vi "Receiver_Example - 1 Channel_Control.vi"() -> ()   [LabVIEW 2022 SP3]
panel:
  out "Numeric":dbl
  out "Iterations 2":i32
  in  "OFDM - 4QAM/16QAM":bool
  out "Error out 2":errorcluster
  in  "Tab Control 2":enum32{"OFDM - 4QAM", "16QAM"}(tab)
  in  "Tab Control":enum32{"USRP Parameters", "Rx Info", "BER"}(tab)
  in  "USRP ControledParameters":T1={"Active Antenna"="RX2", "Gain (dB)"=10.0, "Carrier Frequency"=2400000000.0, "IQ Rate"=2000000.0, "Active channels"="0"} {"IQ Rate" format="%#_6p"; "Carrier Frequency" format="%#_6p"; "Gain (dB)" format="%#_6f"}
  in  "Device selection":refnum<k15>="RIO0"
  in  "Trigger level":dbl=0.005 format="%f"
  out "?":T2
  out "SIG valid?":bool
  out "Frequency offset":dbl
  out "Coerced Parameters":T3={"IQ Rate"=100000.0, "Carrier  Freq."=100000.0, "Gain"=0.0} {"Gain" format="%#_6f"; "Carrier  Freq." format="%#_6p"; "IQ Rate" format="%#_6p"}
  out "Error out":errorcluster
  in  "Boolean":bool
  in  "Expected message LP":string="Non Critical Data\nNon Critical Data\nNon Critical Data\nNon Critical Data\nNon Critical Data"
  in  "Record BER":bool
  in  "Refresh Button":bool
  out "Inst. BER LP":dbl format="%#_4g"
  out "No. Bits LP":dbl
  out "Acum. Err LP":dbl
  out "Acc. BER LP":dbl format="%#_4g"
  in  "Expected message 2 HP":string="Critical Dataaaaa\nCritical Dataaaaa\nCritical Dataaaaa\nCritical Dataaaaa\nCritical Dataaaaa"
  out "Inst. BER HP":dbl format="%#_4g"
  out "Acum. Err HP":dbl
  out "No. Bits HP":dbl
  out "Acc. BER  HP":dbl format="%#_4g"
  out "Expected message LP Detected":string="Non Critical Data\nNon Critical Data\nNon Critical Data\nNon Critical Data\nNon Critical Data"
  out "Expected message  HP  Detected":string="Critical Dataaaaa\nCritical Dataaaaa\nCritical Dataaaaa\nCritical Dataaaaa\nCritical Dataaaaa"
  in  "Boolean 2":bool
  out "Constellation Map":cdb[](graph)
  out "Low-Power Decoded Message":string
  out "High-Power Decoded Message":string
  out "Low-Power BER Graph":dbl(graph)
  out "High-Power BER Graph":dbl(graph)
  out "Low-Power Instantaneous BER Graph":u8(slide) scale=0.0..100.0
  out "High-Power Instantaneous BER Graph":u8(slide) scale=0.0..100.0
  in  "Low-Power Window Size":dbl=15.0 format="%#_6p"
  in  "High-Power Window Size":dbl=15.0 format="%#_6p"
  out "Reconstructed Image":T4(plugin-control)
  out "Expected message  HP  Detected 2":string="Critical Dataaaaa\nCritical Dataaaaa\nCritical Dataaaaa\nCritical Dataaaaa\nCritical Dataaaaa"
  in  "Boolean 3":bool
  in  "High-Power Window Size 2":dbl=15.0 format="%#_6p"
  out "High-Power Instantaneous BER Graph 2":u8(slide) scale=0.0..100.0
  out "High-Power BER Graph 2":dbl(graph)
  out "No. Bits HP 2":dbl
  out "Acc. BER  HP 2":dbl format="%#_4g"
  out "Acum. Err HP 2":dbl
  out "Inst. BER HP 2":dbl format="%#_4g"
  in  "Expected message 2 HP 2":string="Critical Dataaaaa\nCritical Dataaaaa\nCritical Dataaaaa\nCritical Dataaaaa\nCritical Dataaaaa"
  out "High-Power Decoded Message 2":string
  in  "Record BER 2":bool
  out "Constellation Map 2":cdb[](graph)
  out "Frequency offset 2":dbl
  out "SIG valid? 2":bool
  in  "Refresh Button 2":bool
  out "Reconstructed Image":T4(plugin-control)
  out "Iterations":i32
  in  "error in (no error)":errorcluster
  # "OFDM Superposition Coded Receiver"
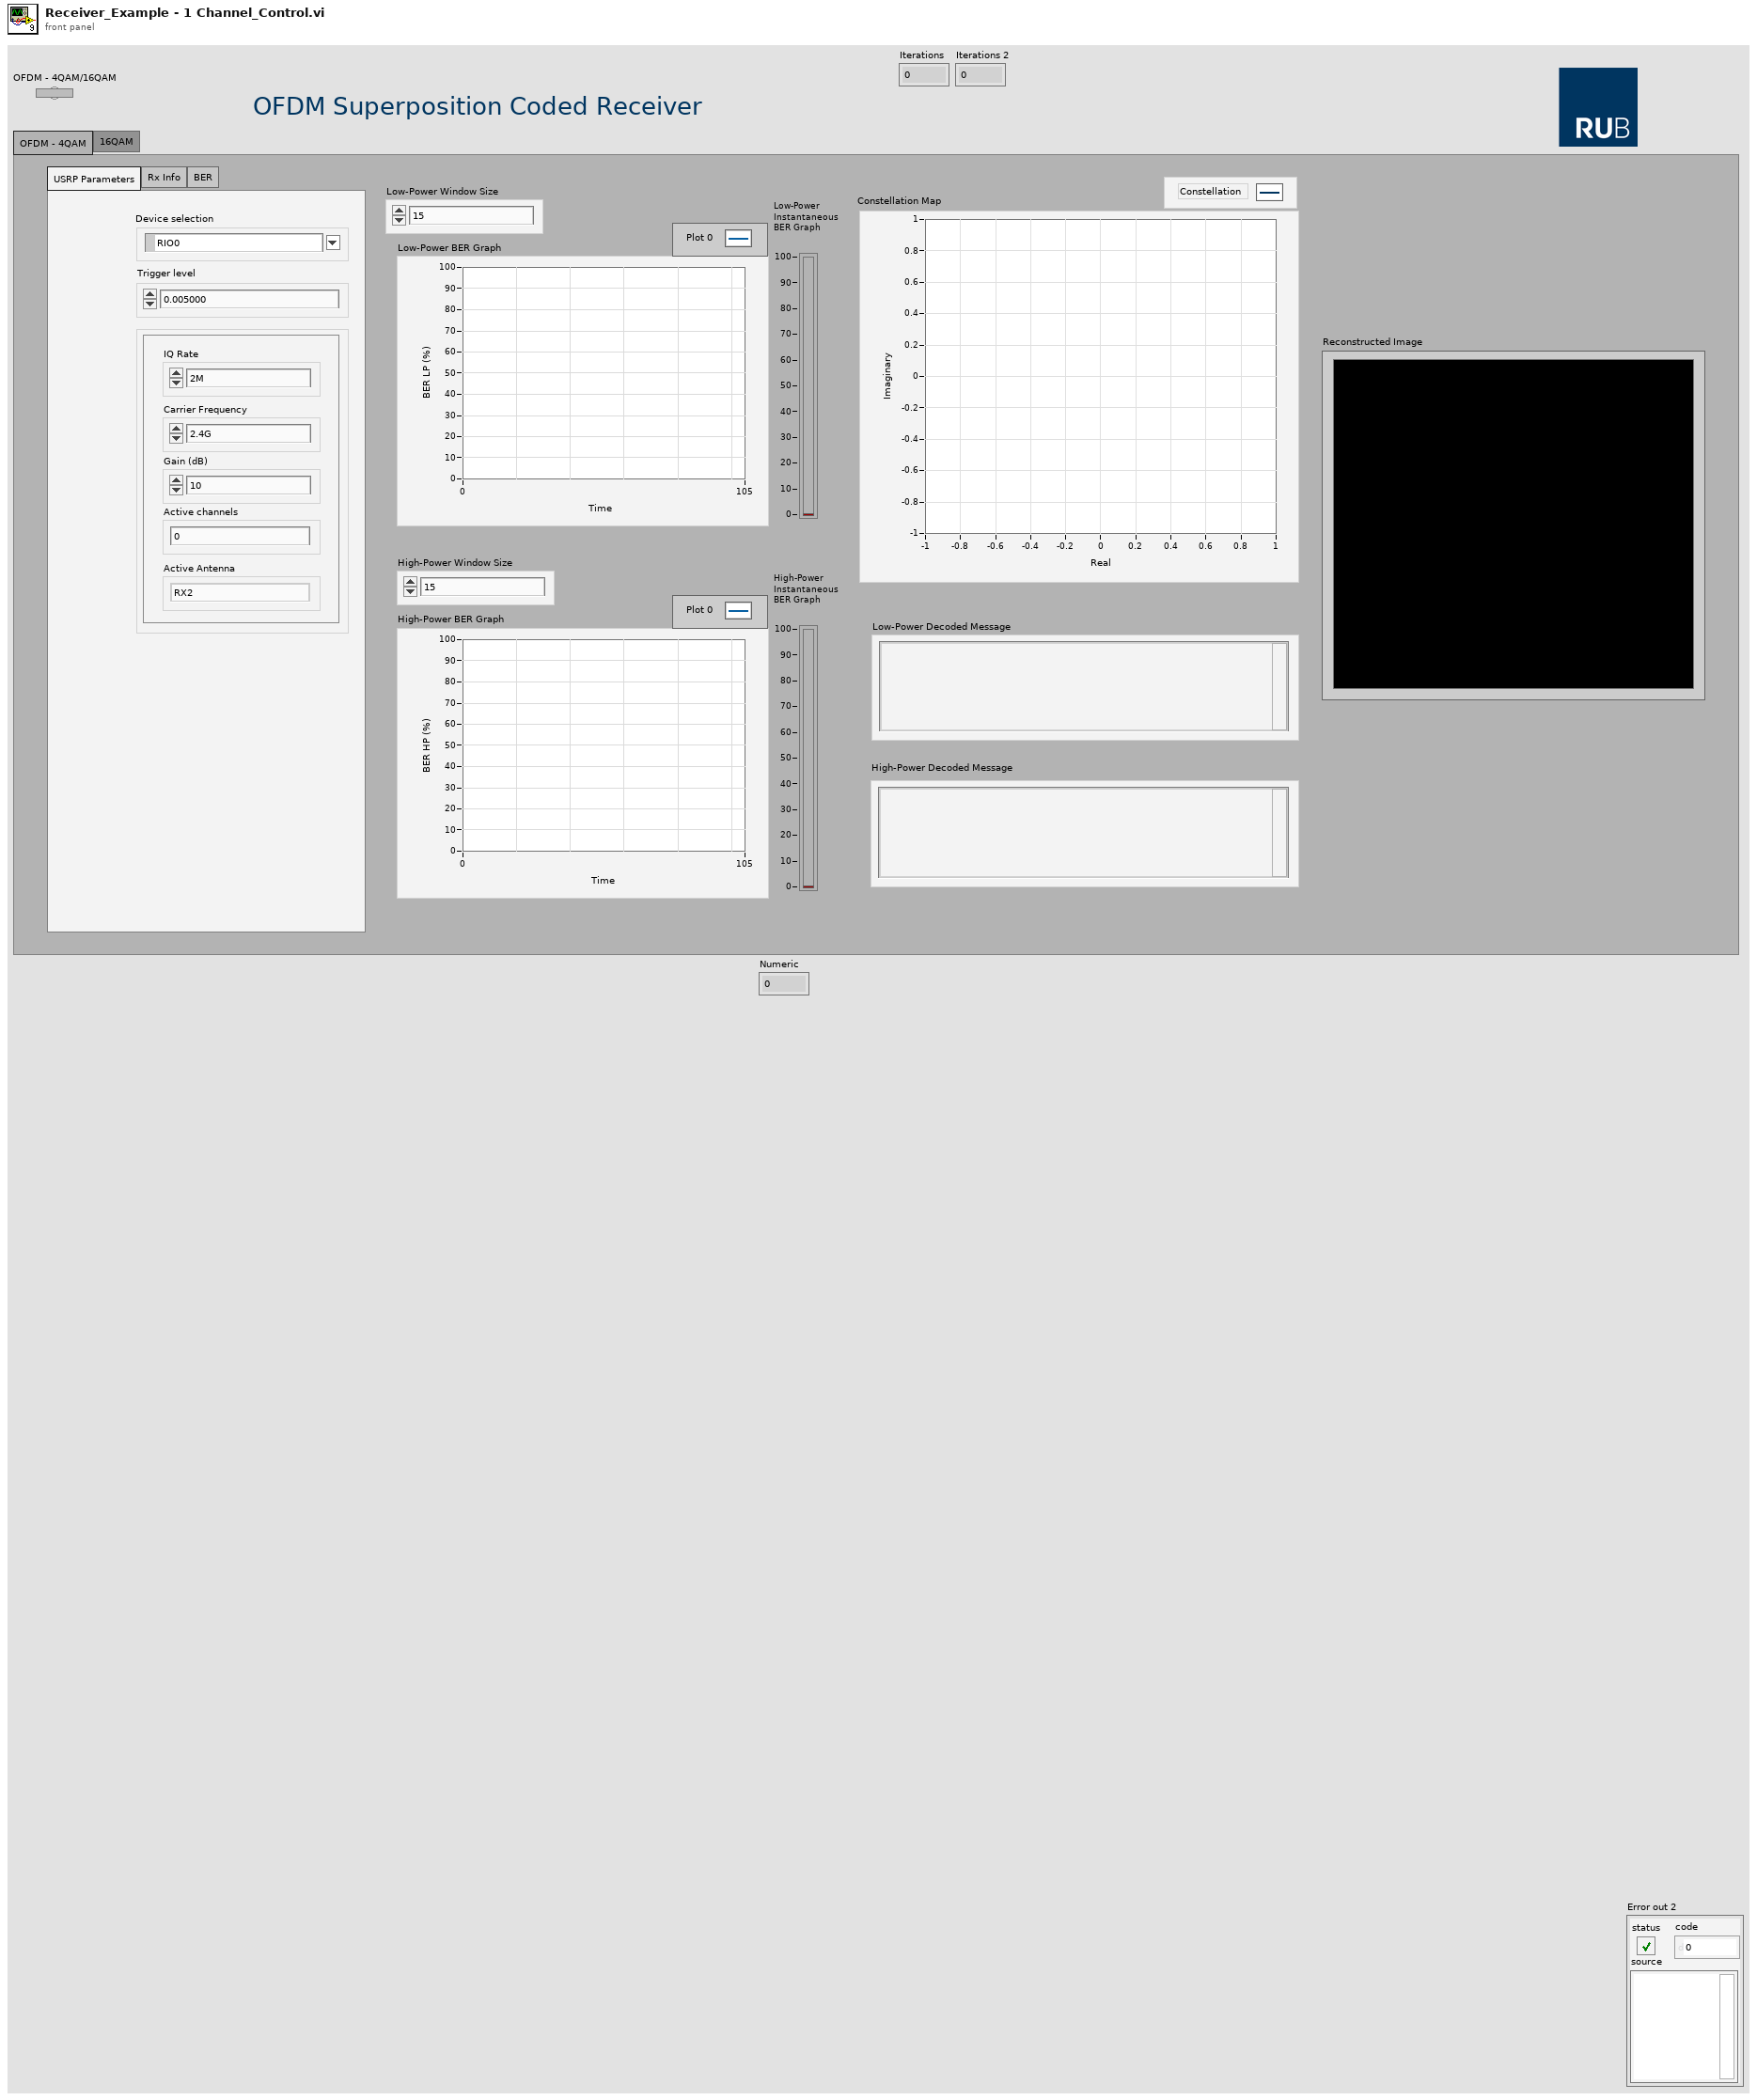
[diagram p1: front panel]
types:
  T1 = cluster{"Active Antenna":string, "Gain (dB)":dbl, "Carrier Frequency":dbl, "IQ Rate":dbl, "Active channels":string}
  T2 = cluster{"Modulation type":enum16{"QPSK(4QAM)", "64QAM", "16QAM", "BPSK"}, "BCC rate (k/n)":enum16{"1/2", "2/3", "3/4"}}
  T3 = cluster{"IQ Rate":dbl, "Carrier  Freq.":dbl, "Gain":dbl}
  T4 = typedef "IMAQ Image.ctl" = refnum<image>
  T5 = cluster{"coerced IQ rate":dbl, "coerced carrier frequency":dbl, "coerced gain":dbl}
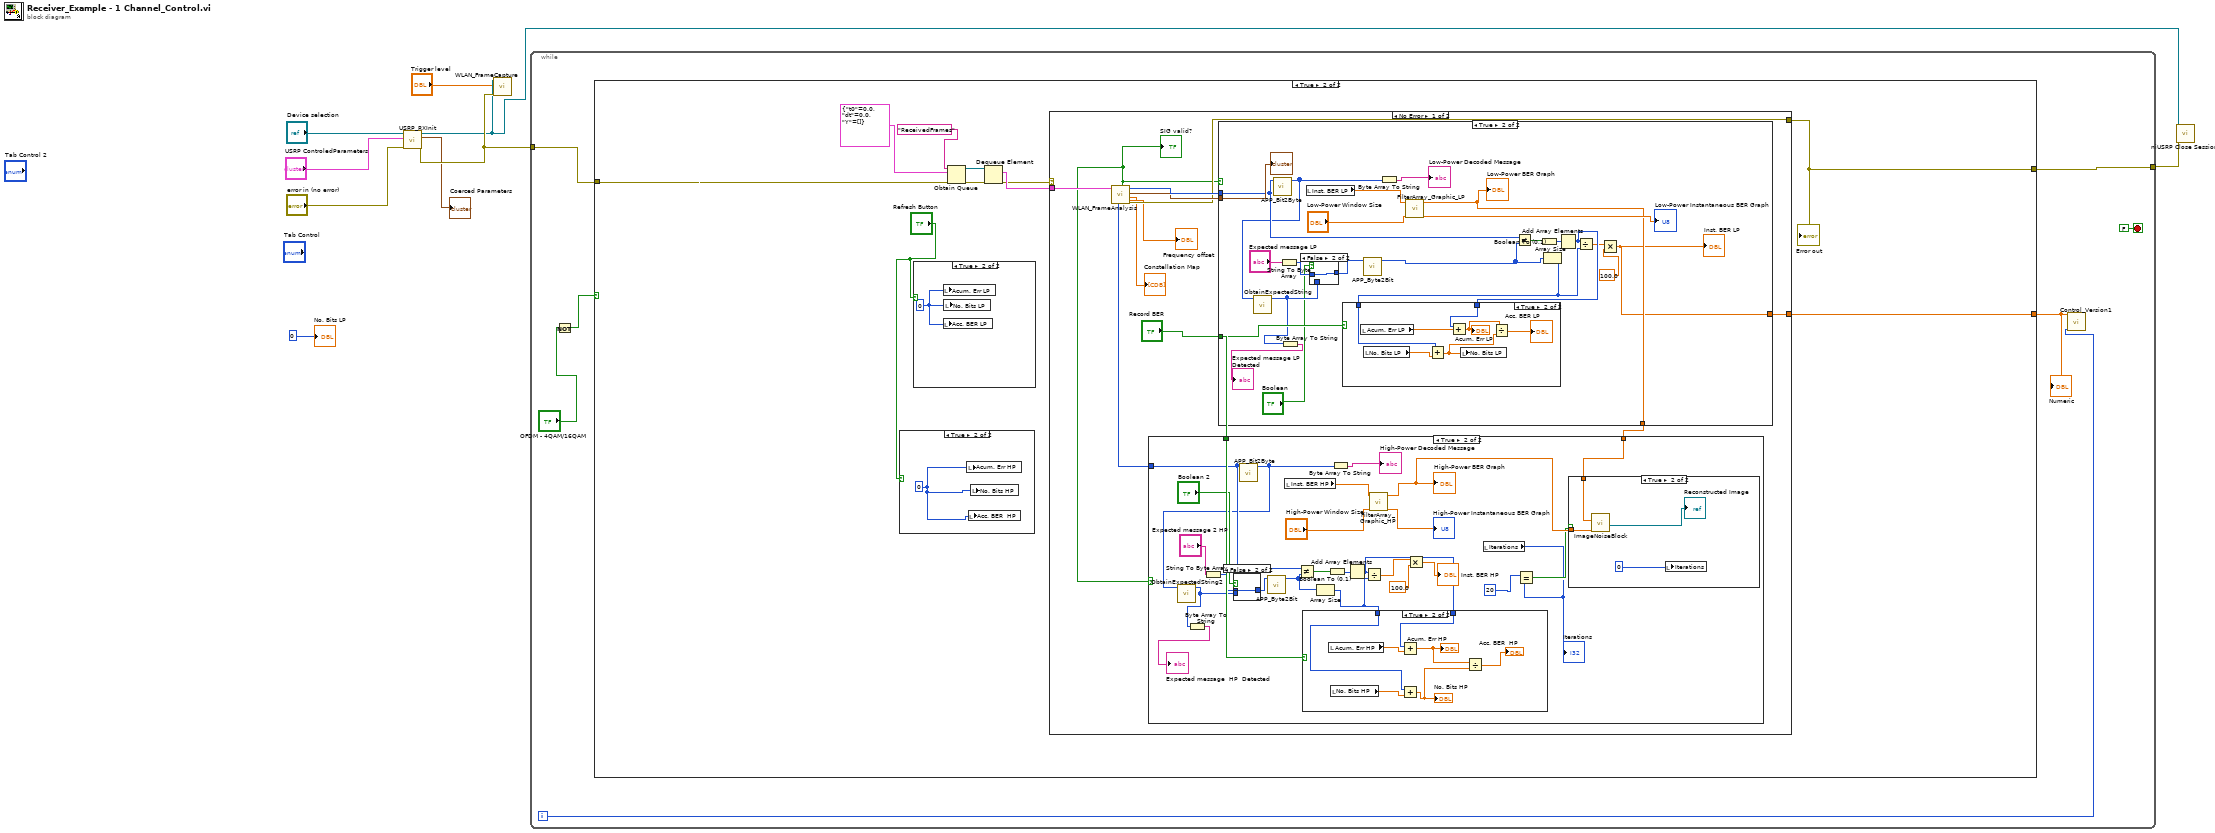
[diagram p0: block diagram]
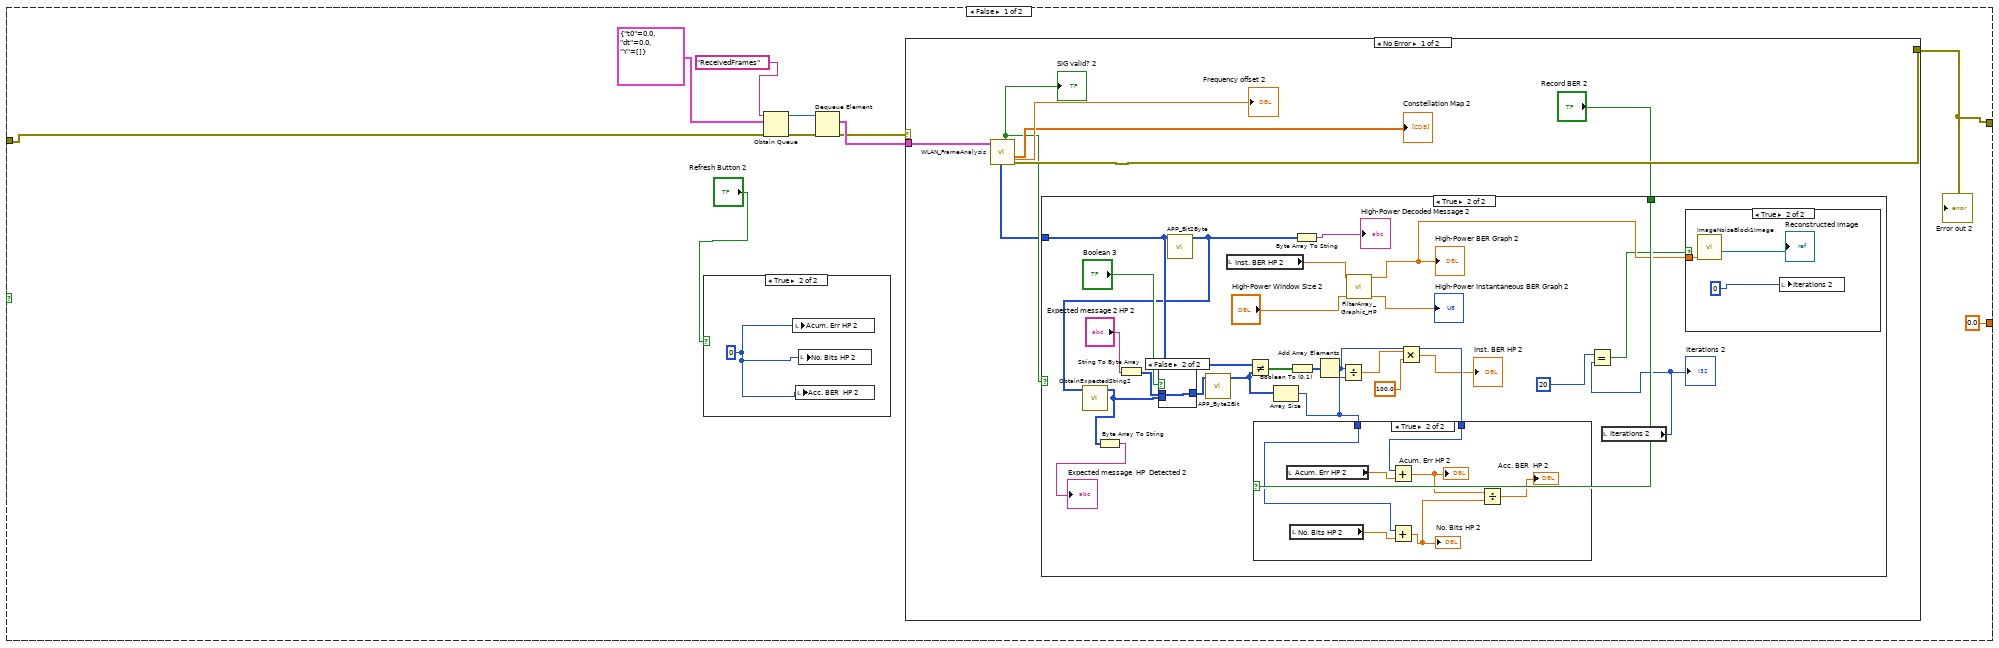
[diagram p2: hidden frame]
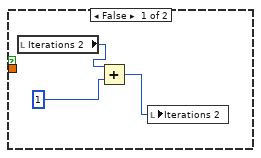
[diagram p5: hidden frame]
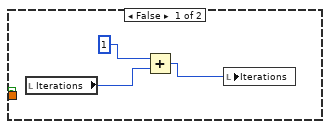
[diagram p13: hidden frame]
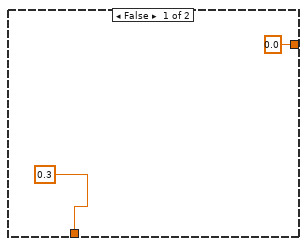
[diagram p15: hidden frame]
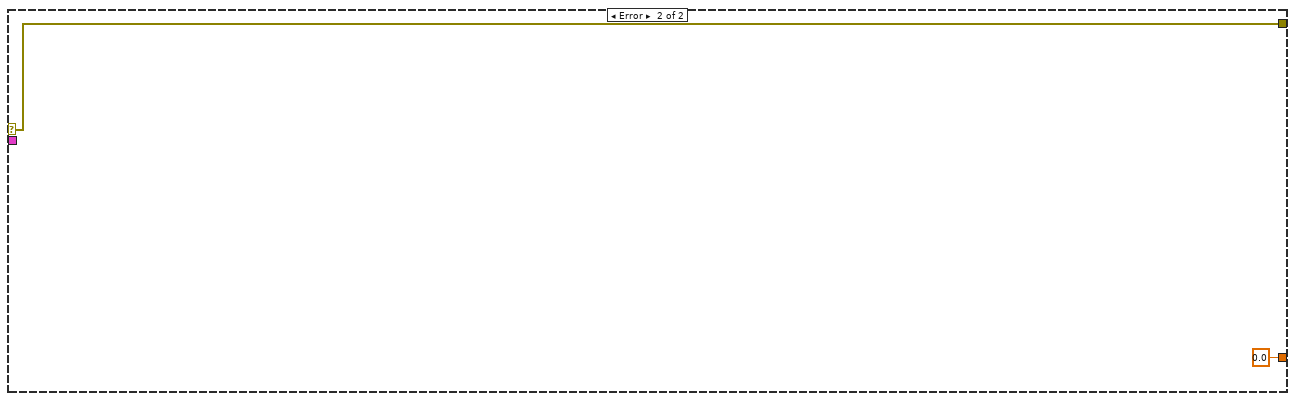
[diagram p18: hidden frame]
diagram:
  n1 = call "USRP_RXInit.vi"("device names"="Device selection", "USRP ControledParameters"="USRP ControledParameters", "error in (no error)"="error in (no error)") -> ("session handle out"=w6:refnum<k15>, "USRP CoercedParamters"=→"Coerced Parameters":T5, "error out"=w8:errorcluster)  [unwired: 5 in]
  n2 = call "WLAN_FrameCapture.vi"("error in (no error)"=w8, "Trigger level"="Trigger level", "session handle"=w6) -> ()  [unwired: 8 in]
  n3 = while {
    tunnel: w8 -> [w16]
    tunnel: [w15] -> w7
    i -> [w10]
    stop <- FALSE stop-if-true
    n4 = Not(x="OFDM - 4QAM/16QAM") -> (.not. x?=w12:bool)
    n5 = case shown="True" w12 {
      tunnel: w16 -> [w19 w78]
      tunnel: [w18 w77] -> w15
      tunnel: [0.0 w76] -> w11
      frame False {
        n6 = case shown="True" "Refresh Button 2" {
          frame False {
          }
          frame True {
            w27 = 0
            n7 = local write "Acum. Err HP 2"(w27) -> ()
            n8 = local write "Acc. BER  HP 2"(w27) -> ()
            n9 = local write "No. Bits HP 2"(w27) -> ()
          }
        }
        n10 = Obtain Queue(name (unnamed)="ReceivedFrames", element data type=cluster{"t0":dbl, "dt":dbl, "Y":cdb[]} {"t0"=0.0, "dt"=0.0, "Y"=[]} ("data"), error in (no error)=w19) -> (queue out=w20:refnum<queue>, error out=w23:errorcluster)  [unwired: 2 in, 1 out]
        n11 = Dequeue Element(queue=w20, error in (no error)=w23) -> (element=w22:cluster{"t0":dbl, "dt":dbl, "Y":cdb[]}, error out=w21:errorcluster)  [unwired: 1 in, 2 out]
        n12 = case shown="No Error" w21 {
          selector: w21 -> [_ w75]
          tunnel: w22 -> [w33 _]
          tunnel: [w34 w75] -> w18
          frame No Error {
            n13 = call "WLAN_FrameAnalysis.vi"("input cluster"=w33) -> ("error out"=w34:errorcluster, "Constellation"=→"Constellation Map 2":cdb[], "Frequency offset"=→"Frequency offset 2":dbl, "SIG valid?"=w29:bool, "outputbitsHP"=w28:i8[])  [unwired: 4 in, 2 out]
            "SIG valid? 2" <- w29
            n14 = case shown="True" w29 {
              tunnel: "Record BER 2" -> [_ w53]
              tunnel: w28 -> [_ w48]
              frame False {
              }
              frame True {
                n15 = String To Byte Array(string="Expected message 2 HP 2") -> (unsigned byte array=w46:u8[])
                n16 = call "APP_Bit2Byte.vi"("input bit stream"=w48) -> ("output byte stream"=w42:u8[])  [unwired: 10 in]
                n17 = call "ObtainExpectedString2.vi"("Array"=w42) -> ("detectedMessage"=w44:i8[])  [unwired: 9 in]
                n18 = Byte Array To String(unsigned byte array=w44) -> (string=→"Expected message  HP  Detected 2":string)
                n19 = case shown="False" "Boolean 3" {
                  tunnel: [w66 w67] -> w47
                  tunnel: w46 -> [_ w67]
                  tunnel: w44 -> [w66 _]
                  frame True {
                  }
                  frame False {
                  }
                }
                n20 = call "APP_Byte2Bit.vi"("input byte stream"=w47) -> ("output bit stream"=w49:i8[])  [unwired: 10 in]
                n21 = local read "Inst. BER HP 2"() -> (w52:dbl)
                n22 = Not Equal?(x=w48, y=w49) -> (x != y?=w57:bool[])
                n23 = Array Size(array=w49) -> (size(s)=w54:i32)
                n24 = Boolean To (0,1)(Boolean=w57) -> (0, 1=w56:i16[])
                n25 = Byte Array To String(unsigned byte array=w42) -> (string=→"High-Power Decoded Message 2":string)
                n26 = Add Array Elements(numeric array=w56) -> (sum=w55:i16)
                n27 = case shown="True" w53 {
                  tunnel: w55 -> [_ w73]
                  tunnel: w54 -> [_ w68]
                  frame False {
                  }
                  frame True {
                    n28 = local read "Acum. Err HP 2"() -> (w74:dbl)
                    n29 = local read "No. Bits HP 2"() -> (w70:dbl)
                    n30 = Add(x=w73, y=w74) -> (x+y=w72:dbl)
                    "Acum. Err HP 2" <- w72
                    n31 = Add(x=w68, y=w70) -> (x+y=w69:dbl)
                    "No. Bits HP 2" <- w69
                    n32 = Divide(x=w72, y=w69) -> (x/y=→"Acc. BER  HP 2":dbl)
                  }
                }
                n33 = Divide(x=w55, y=w54) -> (x/y=w41:dbl)
                n34 = call "FilterArray_Graphic_HP.vi"("Window Size"="High-Power Window Size 2", "Instantaneous BER"=w52) -> ("Slide Bar"=→"High-Power Instantaneous BER Graph 2":dbl, "Graph Instantaneous BER"=w38:dbl)  [unwired: 4 in]
                "High-Power BER Graph 2" <- w38
                n35 = Multiply(x=w41, y=100.0) -> (x*y=→"Inst. BER HP 2":dbl)
                n36 = local read "Iterations 2"() -> (w36:i32)
                "Iterations 2" <- w36
                n37 = Equal?(x=20, y=w36) -> (x = y?=w35:bool)
                n38 = case shown="True" w35 {
                  tunnel: w38 -> [_ w65]
                  frame False {
                    n39 = local read "Iterations 2"() -> (w62:i32)
                    n40 = Add(x=w62, y=1) -> (x+y=w60:i32)
                    n41 = local write "Iterations 2"(w60) -> ()
                  }
                  frame True {
                    n42 = call "ImageNoiseBlock1Image.vi"("BERHP"=w65) -> ("High-Power Image"=→"Reconstructed Image":T4)  [unwired: 9 in]
                    n43 = local write "Iterations 2"(0) -> ()
                  }
                }
              }
            }
          }
          frame Error {
          }
        }
        "Error out 2" <- w18
      }
      frame True {
        n44 = case shown="True" "Refresh Button" {
          frame False {
          }
          frame True {
            w86 = 0
            n45 = local write "Acum. Err HP"(w86) -> ()
            n46 = local write "Acc. BER  HP"(w86) -> ()
            n47 = local write "No. Bits HP"(w86) -> ()
          }
        }
        n48 = case shown="True" "Refresh Button" {
          frame False {
          }
          frame True {
            w87 = 0
            n49 = local write "Acum. Err LP"(w87) -> ()
            n50 = local write "Acc. BER LP"(w87) -> ()
            n51 = local write "No. Bits LP"(w87) -> ()
          }
        }
        n52 = Obtain Queue(name (unnamed)="ReceivedFrames", element data type=cluster{"t0":dbl, "dt":dbl, "Y":cdb[]} {"t0"=0.0, "dt"=0.0, "Y"=[]} ("data"), error in (no error)=w78) -> (queue out=w79:refnum<queue>, error out=w82:errorcluster)  [unwired: 2 in, 1 out]
        n53 = Dequeue Element(queue=w79, error in (no error)=w82) -> (element=w81:cluster{"t0":dbl, "dt":dbl, "Y":cdb[]}, error out=w80:errorcluster)  [unwired: 1 in, 2 out]
        n54 = case shown="No Error" w80 {
          selector: w80 -> [_ w176]
          tunnel: w81 -> [w95 _]
          tunnel: [w96 w176] -> w77
          tunnel: [w88 0.0] -> w76
          frame No Error {
            n55 = call "WLAN_FrameAnalysis.vi"("input cluster"=w95) -> ("error out"=w96:errorcluster, "Constellation"=→"Constellation Map":cdb[], "Modulation parameter"=w97:T2, "output bits"=w98:i8[], "Frequency offset"=→"Frequency offset":dbl, "SIG valid?"=w91:bool, "outputbitsHP"=w90:i8[])  [unwired: 4 in]
            "SIG valid?" <- w91
            n56 = case shown="True" w91 {
              tunnel: w98 -> [_ w150]
              tunnel: w97 -> [_ w165]
              tunnel: "Record BER" -> [_ w159]
              tunnel: [0.3 ("Graph Instantaneous BER") w155] -> w89
              tunnel: [0.0 w143] -> w88
              frame False {
              }
              frame True {
                n57 = call "APP_Bit2Byte.vi"("input bit stream"=w150) -> ("output byte stream"=w146:u8[])  [unwired: 10 in]
                n58 = call "ObtainExpectedString.vi"("Array"=w146) -> ("detectedMessage"=w148:i8[])  [unwired: 9 in]
                n59 = String To Byte Array(string="Expected message LP") -> (unsigned byte array=w151:u8[])
                n60 = Byte Array To String(unsigned byte array=w148) -> (string=→"Expected message LP Detected":string)
                n61 = local read "Inst. BER LP"() -> (w158:dbl)
                n62 = case shown="False" "Boolean" {
                  tunnel: [w166 w167] -> w152
                  tunnel: w151 -> [_ w167]
                  tunnel: w148 -> [w166 _]
                  frame True {
                  }
                  frame False {
                  }
                }
                n63 = call "APP_Byte2Bit.vi"("input byte stream"=w152) -> ("output bit stream"=w153:i8[])  [unwired: 10 in]
                n64 = Byte Array To String(unsigned byte array=w146) -> (string=→"Low-Power Decoded Message":string)
                n65 = call "FilterArray_Graphic_LP.vi"("Window Size"="Low-Power Window Size", "Instantaneous BER"=w158) -> ("Slide Bar"=→"Low-Power Instantaneous BER Graph":dbl, "Graph Instantaneous BER"=w155:dbl)  [unwired: 4 in]
                "Low-Power BER Graph" <- w155
                n66 = Not Equal?(x=w150, y=w153) -> (x != y?=w161:bool[])
                n67 = Boolean To (0,1)(Boolean=w161) -> (0, 1=w154:i16[])
                n68 = Array Size(array=w153) -> (size(s)=w163:i32)
                n69 = Add Array Elements(numeric array=w154) -> (sum=w160:i16)
                n70 = case shown="True" w159 {
                  tunnel: w163 -> [_ w173]
                  tunnel: w160 -> [_ w171]
                  frame False {
                  }
                  frame True {
                    n71 = local read "Acum. Err LP"() -> (w172:dbl)
                    n72 = local read "No. Bits LP"() -> (w174:dbl)
                    n73 = Add(x=w173, y=w174) -> (x+y=w168:dbl)
                    n74 = Add(x=w171, y=w172) -> (x+y=w170:dbl)
                    "Acum. Err LP" <- w170
                    n75 = local write "No. Bits LP"(w168) -> ()
                    n76 = Divide(x=w170, y=w168) -> (x/y=→"Acc. BER LP":dbl)
                  }
                }
                n77 = Divide(x=w160, y=w163) -> (x/y=w145:dbl)
                n78 = Multiply(x=w145, y=100.0) -> (x*y=w143:dbl)
                "Inst. BER LP" <- w143
                "?" <- w165
              }
            }
            n79 = case shown="True" w91 {
              tunnel: "Record BER" -> [_ w118]
              tunnel: w90 -> [_ w108]
              tunnel: w89 -> [_ w113]
              frame False {
              }
              frame True {
                n80 = String To Byte Array(string="Expected message 2 HP") -> (unsigned byte array=w106:u8[])
                n81 = call "APP_Bit2Byte.vi"("input bit stream"=w108) -> ("output byte stream"=w102:u8[])  [unwired: 10 in]
                n82 = call "ObtainExpectedString2.vi"("Array"=w102) -> ("detectedMessage"=w104:i8[])  [unwired: 9 in]
                n83 = Byte Array To String(unsigned byte array=w104) -> (string=→"Expected message  HP  Detected":string)
                n84 = case shown="False" "Boolean 2" {
                  tunnel: [w125 w126] -> w107
                  tunnel: w106 -> [_ w126]
                  tunnel: w104 -> [w125 _]
                  frame True {
                  }
                  frame False {
                  }
                }
                n85 = call "APP_Byte2Bit.vi"("input byte stream"=w107) -> ("output bit stream"=w112:i8[])  [unwired: 10 in]
                n86 = local read "Inst. BER HP"() -> (w117:dbl)
                n87 = Not Equal?(x=w108, y=w112) -> (x != y?=w122:bool[])
                n88 = Array Size(array=w112) -> (size(s)=w119:i32)
                n89 = Boolean To (0,1)(Boolean=w122) -> (0, 1=w121:i16[])
                n90 = Byte Array To String(unsigned byte array=w102) -> (string=→"High-Power Decoded Message":string)
                n91 = Add Array Elements(numeric array=w121) -> (sum=w120:i16)
                n92 = case shown="True" w118 {
                  tunnel: w120 -> [_ w139]
                  tunnel: w119 -> [_ w134]
                  frame False {
                  }
                  frame True {
                    n93 = local read "Acum. Err HP"() -> (w140:dbl)
                    n94 = local read "No. Bits HP"() -> (w136:dbl)
                    n95 = Add(x=w139, y=w140) -> (x+y=w138:dbl)
                    "Acum. Err HP" <- w138
                    n96 = Add(x=w134, y=w136) -> (x+y=w135:dbl)
                    "No. Bits HP" <- w135
                    n97 = Divide(x=w138, y=w135) -> (x/y=→"Acc. BER  HP":dbl)
                  }
                }
                n98 = Divide(x=w120, y=w119) -> (x/y=w101:dbl)
                n99 = call "FilterArray_Graphic_HP.vi"("Window Size"="High-Power Window Size", "Instantaneous BER"=w117) -> ("Slide Bar"=→"High-Power Instantaneous BER Graph":dbl, "Graph Instantaneous BER"=w114:dbl)  [unwired: 4 in]
                "High-Power BER Graph" <- w114
                n100 = Multiply(x=w101, y=100.0) -> (x*y=→"Inst. BER HP":dbl)
                n101 = local read "Iterations"() -> (w110:i32)
                "Iterations" <- w110
                n102 = Equal?(x=20, y=w110) -> (x = y?=w111:bool)
                n103 = case shown="True" w111 {
                  tunnel: w114 -> [_ w133]
                  tunnel: w113 -> [_ w132]
                  frame False {
                    n104 = local read "Iterations"() -> (w127:i32)
                    n105 = Add(x=1, y=w127) -> (x+y=w128:i32)
                    n106 = local write "Iterations"(w128) -> ()
                  }
                  frame True {
                    n107 = call "ImageNoiseBlock.vi"("BERLP"=w132, "BERHP"=w133) -> ("High-Power Image"=→"Reconstructed Image":T4)  [unwired: 8 in]
                    n108 = local write "Iterations"(0) -> ()
                  }
                }
              }
            }
          }
          frame Error {
          }
        }
        "Error out" <- w77
      }
    }
    "Numeric" <- w11
    n109 = call "Control_Version1.vi"("it"=w10, "BER"=w11) -> ()  [unwired: 10 in]
  }
  n110 = call <instrlib>:"niUSRP Close Session.vi"("session handle"=w6, "error in (no error)"=w7) -> ()  [unwired: 13 in, 1 out]
  "No. Bits LP" <- 0
